vi "Encode.vi"(8 "error in (no error)":errorcluster, 11 "ISO 14443 A DOWN in":refnum<class "ISO 14443 A DOWN.lvclass">) -> (0 "error out":errorcluster, 3 "ISO 14443 A DOWN out":refnum<class "ISO 14443 A DOWN.lvclass">)   [LabVIEW 2019, in "ISO 14443 A DOWN.lvclass"]
uses:
  ISO 14443 A DOWN.lvclass
  TypeDef/Store.ctl
  ISO 14443 A DOWN.lvclass/ISO 14443 A DOWN.ctl
  RFID system.lvclass
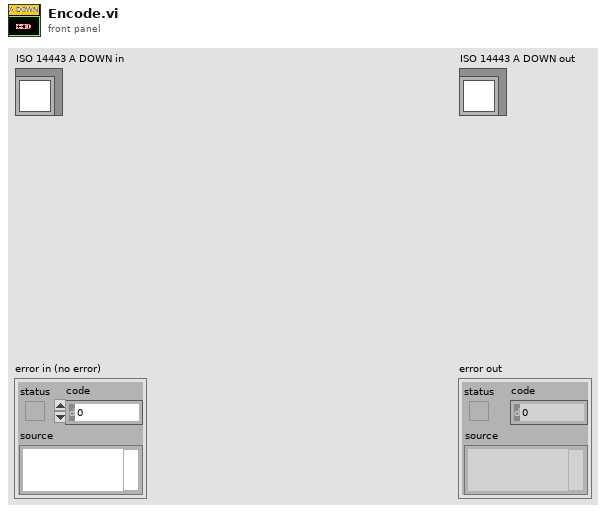
[diagram p1: front panel]
types:
  T1 = typedef "Store.ctl" = enum16{"envelope", "noise", "demSubCar", "CH_frame", "Decode", "demodulate", "in", "out", "sum", "subCarrier", "frame", "command", "encode", "modulate", "encode_UP", "modulate_up", "demod_up", "envelop_up", "sum_up", "out_up", "in_up"}
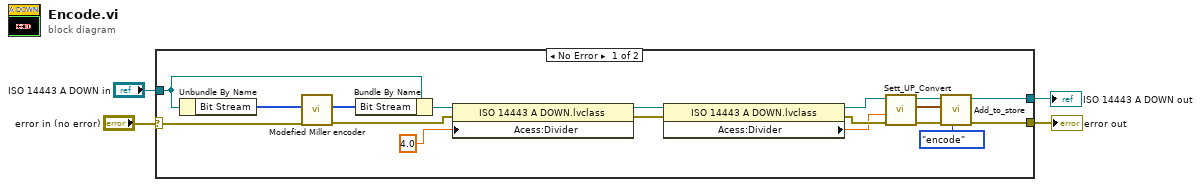
[diagram p0: block diagram]
diagram:
  n1 = case shown="No Error" "error in (no error)" {
    selector: "error in (no error)" -> [w22 w23]
    tunnel: [w13 w23] -> w3
    tunnel: [w16 w24] -> w1
    tunnel: "ISO 14443 A DOWN in" -> [w21 w24]
    frame No Error {
      n2 = Unbundle By Name(w21) -> ("Bit Stream"=w20:u8[])
      n3 = call "Modefied Miller encoder.vi"("Error In"=w22, "Bit stream in"=w20) -> ("error out"=w8:errorcluster, "Bit stream out (NRZ encode)"=w19:u8[])  [unwired: 8 in]
      n4 = Bundle By Name(cluster=w21, "Bit Stream"=w19) -> (w18:refnum<class "ISO 14443 A DOWN.lvclass">)
      n5 = property class="ISO 14443 A DOWN.lvclass"(reference=w18, error in=w8, "Acess:Divider"=4.0 ("Divider")) -> (reference out=w11:refnum<class "ISO 14443 A DOWN.lvclass">, error out=w7:errorcluster)
      n6 = property class="ISO 14443 A DOWN.lvclass"(reference=w11, error in=w7) -> (reference out=w10:refnum<class "ISO 14443 A DOWN.lvclass">, error out=w6:errorcluster, "Acess:Divider"=w5:dbl)
      n7 = call-dynamic "Sett_UP_Convert.vi"("error in (no error)"=w6, "Divider(1)"=w5, "ISO 14443 A DOWN in"=w10) -> ("error out"=w14:errorcluster, "Waveform"=w15:waveform(dbl), "ISO 14443 A DOWN out"=w17:refnum<class "ISO 14443 A DOWN.lvclass">)  [unwired: 6 in]
      n8 = call "Add_to_store.vi"("Store"=Store."encode", "error in (no error)"=w14, "Waveform"=w15, "RFID system in"=w17) -> ("error out"=w13:errorcluster, "RFID system out"=w16:refnum<class "ISO 14443 A DOWN.lvclass">)  [unwired: 6 in]
    }
    frame Error {
    }
  }
  "error out" <- w3
  "ISO 14443 A DOWN out" <- w1
